vi "Set Source Preference.vi"(8 "error in (no error)":errorcluster, 10 "Source Preference (1: 5500A Calibrator)":u32(ring)=1 items=["5725A Amplifier", "5500A Calibrator"], 11 "VISA resource name":refnum<visa-resource-name>) -> (0 "error out":errorcluster, 3 "VISA resource name out":refnum<visa-resource-name>)   [LabVIEW 2013, in "Fluke 5XXX Series Multicalibrators.lvlib"]
doc: "This VI set the source preference to 5500A Calibrator or 5725A Amplifier, when a 5725A Amplifier is attached, which is saved in the 5500A nonvolatile memory. (While saving configuration data in the non-volatile memory, a period of about 2 seconds, the 5500A does not respond to remote commands.) Source preference is used when an output value is programmed to a value that can be sourced by both the 5500A Calibrator and the 5725A Amplifier.\n\nNote:\n\nThis VI is available only for instrument model 5500A with option 5725A."
uses:
  Fluke 5XXX Series Multicalibrators.lvlib
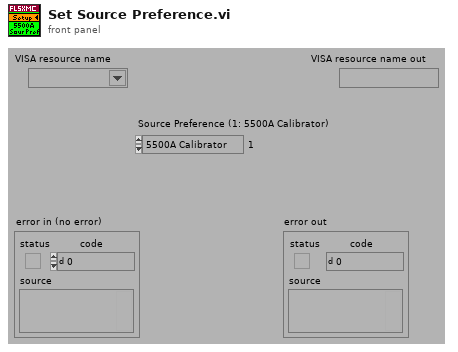
[diagram p1: front panel]
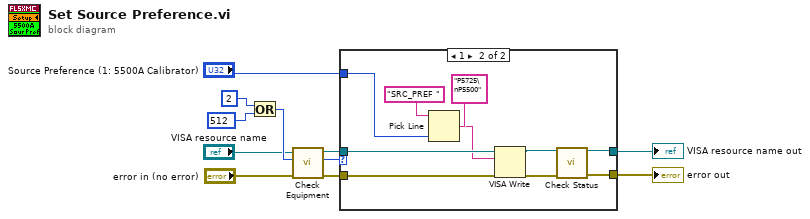
[diagram p0: block diagram]
diagram:
  n1 = Or(x=2 ("Numeric"), y=512 ("Numeric")) -> (x .or. y?=w11:i32)
  n2 = call "Check Equipment.vi"("error in (no error)"="error in (no error)", "Bit Mask"=w11, "VISA resource name"="VISA resource name") -> ("error out"=w10:errorcluster, "Present?"=w9:u32, "VISA resource name out"=w8:refnum<visa-resource-name>)  [unwired: 6 in]
  n3 = case shown="1" w9 {
    tunnel: "Source Preference (1: 5500A Calibrator)" -> [_ w18]
    tunnel: [w12 w14] -> w4
    tunnel: w10 -> [w13 w21]
    tunnel: w8 -> [w12 w20]
    tunnel: [w13 w17] -> w5
    frame 0, Default {
    }
    frame 1 {
      n4 = Pick Line(string ("")="SRC_PREF " ("Reset Command"), multi-line string="P5725\nP5500", line index=w18) -> (output string=w19:string)
      n5 = VISA Write(VISA resource name=w20, write buffer=w19, error in (no error)=w21) -> (VISA resource name out=w15:refnum<visa-resource-name>, error out=w16:errorcluster)  [unwired: 1 out]
      n6 = call "Check Status.vi"("VISA resource name"=w15, "error in (no error)"=w16) -> ("VISA resource name out"=w14:refnum<visa-resource-name>, "error out"=w17:errorcluster)  [unwired: 12 in]
    }
  }
  "VISA resource name out" <- w4
  "error out" <- w5
